vi "xiCam - GetNumberDevices.vi"(8 "error in (no error)":errorcluster, 11 "xiCam In":refnum<k24>) -> (0 "error out":errorcluster, 3 "xiCam Out":refnum<k24>, 4 "GetNumberDevices":i32)   [LabVIEW 2016]
doc: "Description : Returns the number of all discovered devices.\n\n<b>int GetNumberDevices()</b>"
uses:
  C:/Users/Ries Lab/Documents/Microscope Control from Sheng Account/Microscope-Control/Device Library/Cameras/Ximea/xiLIB_64bit/xiLIB/xiCamLib/API/x64/xiApi.NETX64.dll
  API/x64/xiApi.NETX64.dll
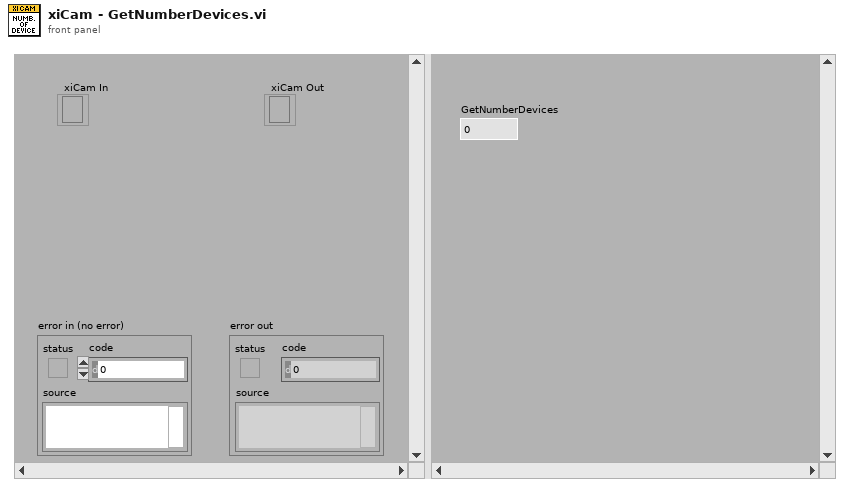
[diagram p1: front panel]
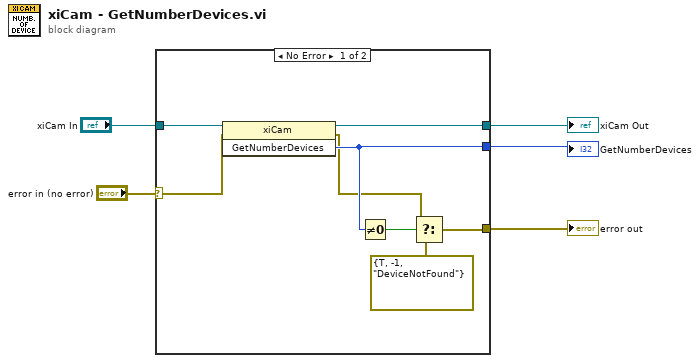
[diagram p0: block diagram]
diagram:
  n1 = case shown="No Error" "error in (no error)" {
    selector: "error in (no error)" -> [w11 w14]
    tunnel: "xiCam In" -> [w13 w15]
    tunnel: [w12 w15] -> w3
    tunnel: [w6 w14] -> w2
    tunnel: [w10 _] -> w1
    frame No Error {
      n2 = invoke class="xiCam" method="GetNumberDevices"(reference=w13, error in=w11) -> (reference out=w12:refnum<k24>, error out=w7:errorcluster, "GetNumberDevices"=w10:i32)  [unwired: 1 in]
      n3 = Not Equal To 0?(x=w10) -> (x != 0?=w9:bool)
      n4 = Select(t=w7, s=w9, f=errorcluster {"status"=TRUE, "code"=-1, "source"="DeviceNotFound"} ("error out")) -> (s? t:f=w6:errorcluster)
    }
    frame Error {
    }
  }
  "error out" <- w2
  "xiCam Out" <- w3
  "GetNumberDevices" <- w1
